vi "GetSnakePosAllCells.vi"(8 "error in (no error)":errorcluster, 11 "Snake in":refnum<class "Snake.lvclass">) -> (0 "error out":errorcluster, 1 "CellPositions":T1[](array[typedef]), 2 "CellColors":u32[](array[numeric]), 3 "Snake out":refnum<class "Snake.lvclass">)   [LabVIEW 2018, in "Snake.lvclass"]
uses:
  Snake.lvclass
  Typedefs/XYposition.ctl
  Snake.lvclass/Snake.ctl
  BodyCell/SnakeBodyCell.lvclass
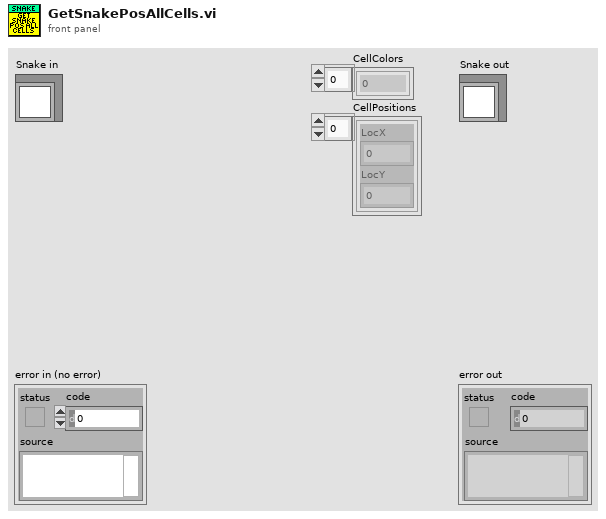
[diagram p1: front panel]
types:
  T1 = typedef "XYposition.ctl" = cluster{"LocX":u16, "LocY":u16}
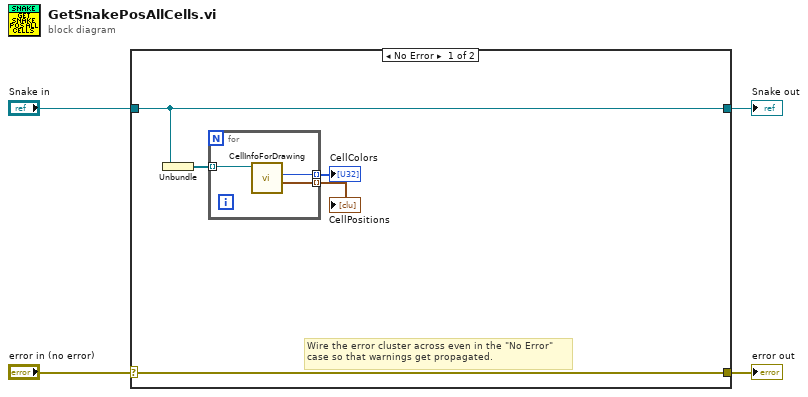
[diagram p0: block diagram]
diagram:
  n1 = case shown="No Error" "error in (no error)" {
    selector: "error in (no error)" -> [w9 w14]
    tunnel: [w9 w14] -> w3
    tunnel: [w8 w13] -> w1
    tunnel: "Snake in" -> [w8 w13]
    frame No Error {
      # "Wire the error cluster across even in the \"No Error\"\ncase so that warnings get propagated."
      n2 = Unbundle(w8) -> (w7:refnum<class "SnakeBodyCell.lvclass">[])
      n3 = for {
        tunnel: w7 -> [w12] mode=indexing
        tunnel: [w11] -> w6 mode=indexing
        tunnel: [w10] -> w5 mode=indexing
        n4 = call "CellInfoForDrawing.vi"("SnakeBodyCell in"=w12) -> ("Position"=w10:T1, "Color"=w11:u32)  [unwired: 7 in, 2 out]
      }
      "CellColors" <- w6
      "CellPositions" <- w5
    }
    frame Error {
    }
  }
  "error out" <- w3
  "Snake out" <- w1
